vi "Find_Beam_Max_Pos.vi"(3 "Mode":T7, 5 "Traverse line In":T4 {"Row Duration (mins)" format="%#.1f"; "Row No" min=0; "Trace Gas Concentration (%)" min=0.0 format="%#.2f"; "Emission Rate (l/min)" format="%#.2f"; "Tunnel Speed" format="%#.2f"; "Start X" format="%#.2f"; "Start Y" format="%#.2f"; "Start Z" format="%#.2f"; "End X" format="%#.2f"; "End Y" format="%#.2f"; "End Z" format="%#.2f"; "Averaging time (min)" min=0.0 format="%#.2f"}) -> (0 "Error Message":string, 1 "Status":T3, 2 "Traverse line Out":T4 {"Row Duration (mins)" format="%#.1f"; "Row No" min=0; "Trace Gas Concentration (%)" min=0.0 format="%#.2f"; "Emission Rate (l/min)" format="%#.2f"; "Tunnel Speed" format="%#.2f"; "Start X" format="%#.2f"; "Start Y" format="%#.2f"; "Start Z" format="%#.2f"; "End X" format="%#.2f"; "End Y" format="%#.2f"; "End Z" format="%#.2f"; "Averaging time (min)" min=0.0 format="%#.2f"})   [LabVIEW 2012]
uses:
  Gen Trav/Traverse_cluster.ctl
  Gen Trav/Spacing.ctl
  Controls/Multi_run_mode.ctl
  Controls/User_Specific_mode.ctl
  Gen Trav/Multi_Run_Status.ctl
  Controls/Beam_Type.ctl
  Gen Trav/Route mapping/Axis.ctl
  ADAM Client/Sub VIs/ADAM Controls/Remember_value_mode.ctl
  Globals/Meas_global.vi
  Utilities/Email_transfer_global.vi
panel:
  out "Picture Log":path
  out "First Call":bool
  out "Fixed Axis":T1
  out "Beams to find":T2[](array[typedef]) items=["Green Unshifted", "Green Shifted", "Blue Unshifted", "Blue Shifted"]
  out "Beam Data":dbl[][](array[numeric]) format="%.2f"
  out "Beam Type":T2 items=["Green Unshifted", "Green Shifted", "Blue Unshifted", "Blue Shifted"]
  # "X                Y                 Z        Datum Power"
  # "Green Unshifted\nGreen Shifted\nBlue Unshifted\nBlue Shifted"
  # "X           Y            Z"
  # "Start"
  # "End"
  # "X           Y            Z"
  # "Start"
  # "End"
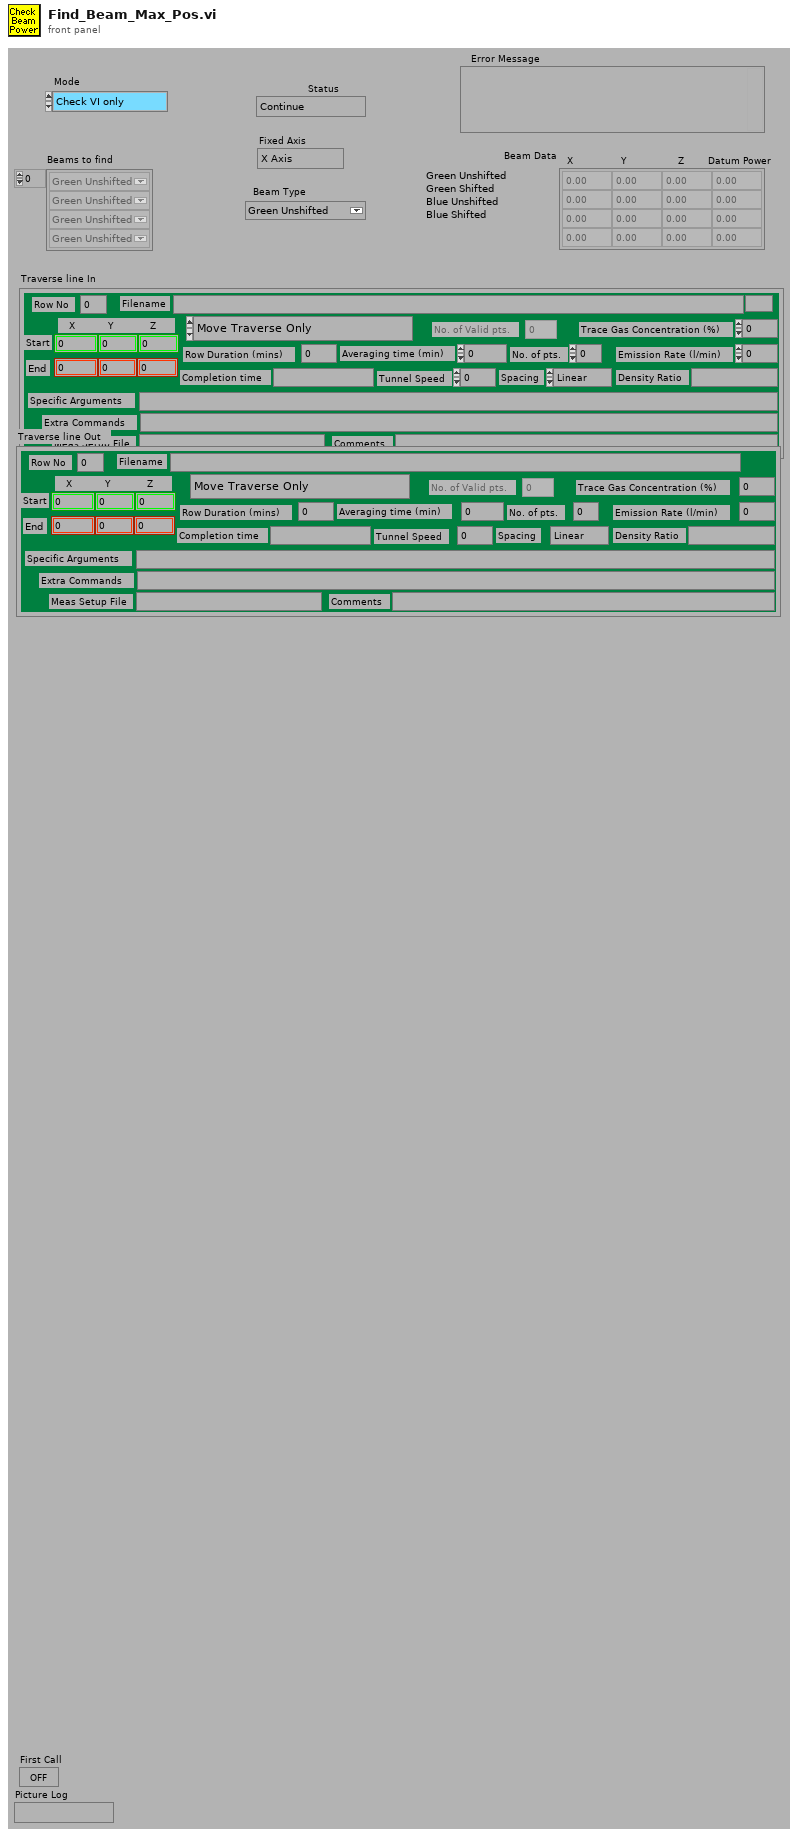
[diagram p1: front panel]
types:
  T1 = typedef "Axis.ctl" = enum16{"X Axis", "X Axis -ve", "Y Axis", "Y Axis -ve", "Z Axis", "Z Axis -ve"}
  T2 = typedef "Beam_Type.ctl" = u16
  T3 = typedef "Multi_Run_Status.ctl" = enum16{"Continue", "Jump to Next Point", "Jump to Next Row", "Jump To Fall Back", "Terminate Run"}
  T4 = typedef "Traverse_cluster.ctl" = cluster{"Start X":dbl, "Start Y":dbl, "Start Z":dbl, "End X":dbl, "End Y":dbl, "End Z":dbl, "No. of pts.":i32, "Spacing":T5, "Filename":path, "Tunnel Speed":dbl, "Averaging time (min)":dbl, "Extra Commands":string, "Specific Arguments":string, "Emission Rate (l/min)":dbl, "Trace Gas Concentration (%)":dbl, "Density Ratio":string, "Comments":string, "Row No":i32, "Row Type Selector":T6, "Completion time":string, "Row Duration (mins)":dbl, "No. of Valid pts.":i32, "Meas Setup File":string}
  T5 = typedef "Spacing.ctl" = enum16{"Linear", "Log", "Gauss", "Specified", "N/A"}
  T6 = typedef "Multi_run_mode.ctl" = enum16{"Move Traverse Only", "Set Tunnel Speed Only", "Set Source Only", "Set Measurement Conditions", "Single Measurement", "Vertical Profile", "Lateral Profile", "Longitudinal Profile", "Explore Volume", "Multi-Axis Profile", "Auto Calibrate", "Meas Fast FID Bkgnd", "Check Beam Power", "Scanning Valve Measurement", "Run VI Named:", "Set ADAM Ch", "Wait (minutes)", "Send Message", "Synchronize With:", "Fall Back to this Row", "Turn Off Row Repeating", "Blank Row", "Traverse 3D Volume"}
  T7 = typedef "User_Specific_mode.ctl" = enum16{"Check VI only", "Run VI"}
  T8 = typedef "LDA_Setup.ctl" = cluster{"dimensions":enum16{"1D", "2D"}, "Analogue Freq Multiplier":dbl}
  T9 = typedef "Remember_value_mode.ctl" = enum16{"Read only", "Read and Write"}
  T10 = enum16{"Load From Excel File", "Save to Excel File"}
  T11 = cluster{"second":i32, "minute":i32, "hour":i32, "day of month":i32, "month":i32, "year":i32, "day of week":i32, "day of year":i32, "is DST":i32}
  T12 = cluster{"path":path, "data":string, "binary":bool, "MIME content-type \n(application/octet-stream)":string}[]
  T13 = cluster{"path":path, "data":string, "binary":bool, "MIME content-type \n(application/octet-stream)":string}
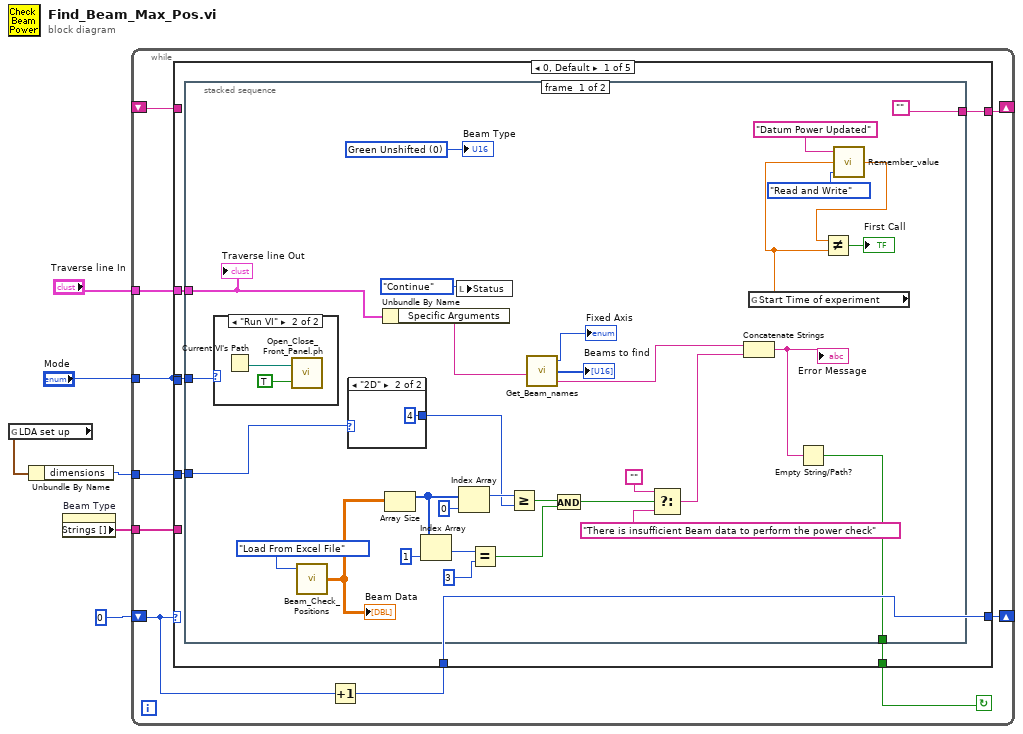
[diagram p0: block diagram]
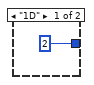
[diagram p2: hidden frame]
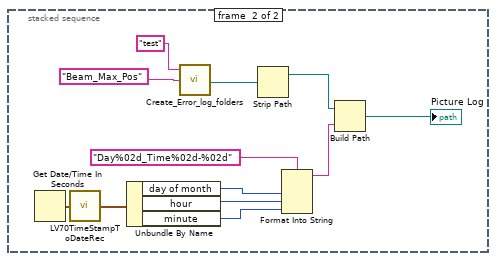
[diagram p4: hidden frame]
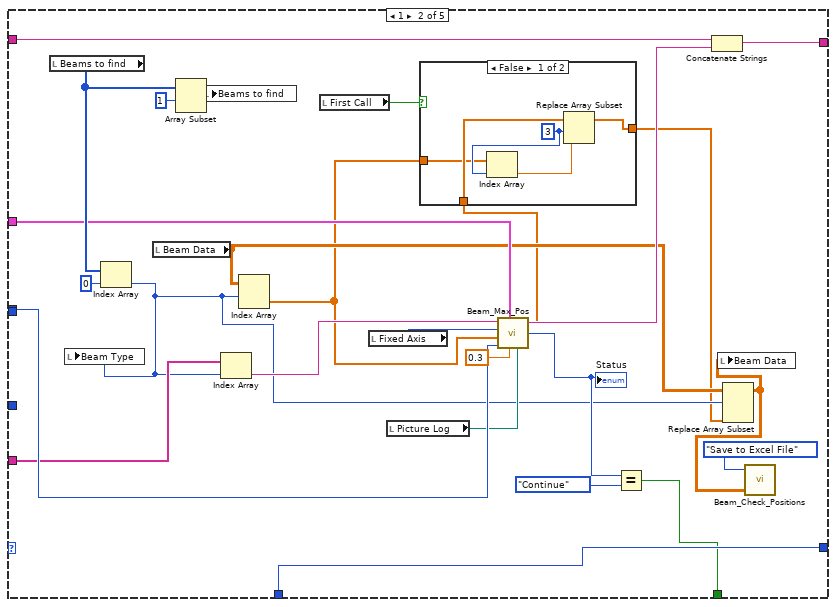
[diagram p5: hidden frame]
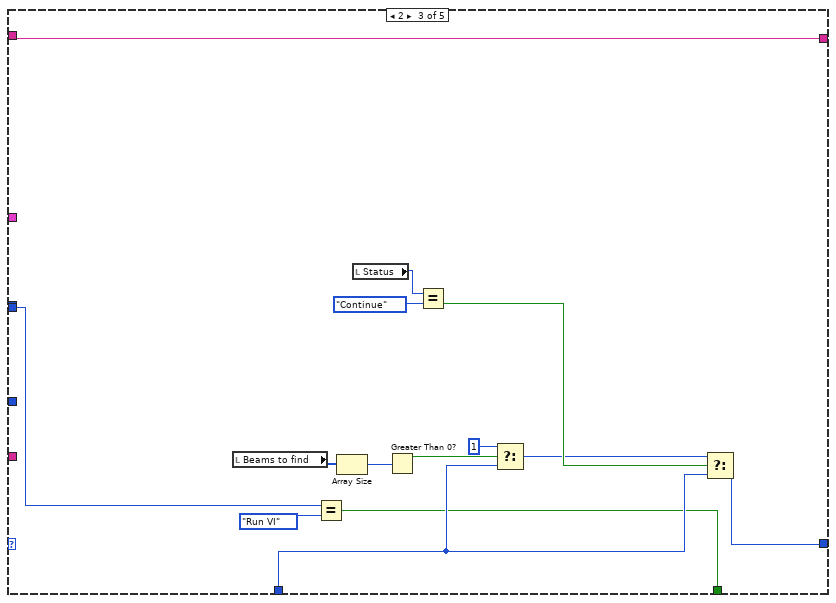
[diagram p7: hidden frame]
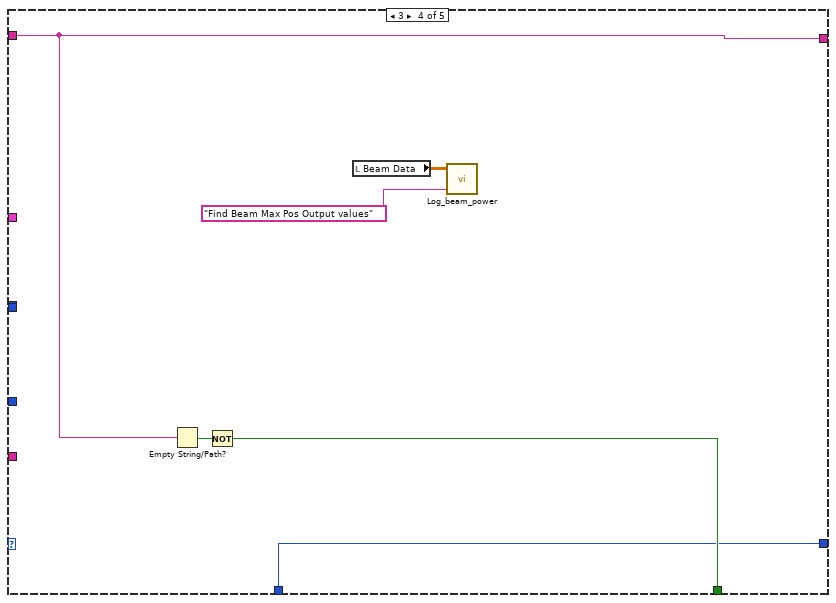
[diagram p8: hidden frame]
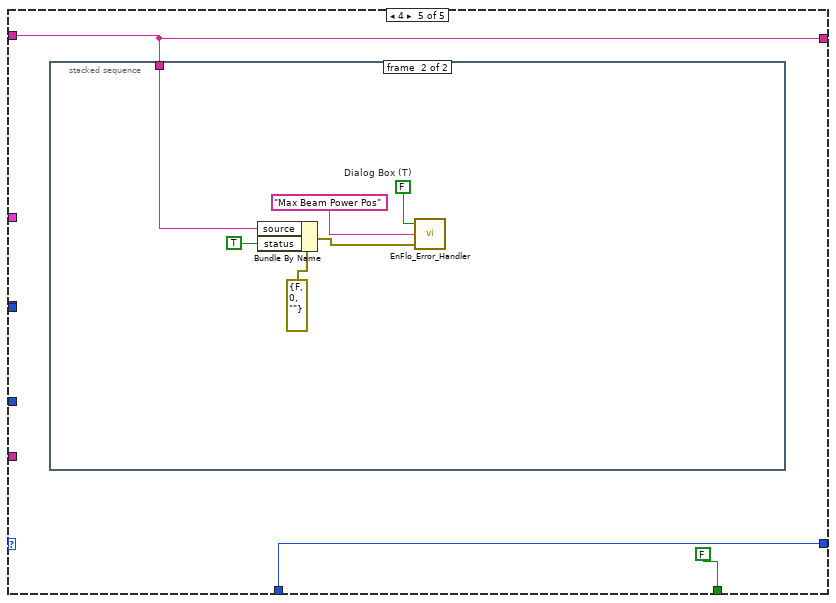
[diagram p9: hidden frame]
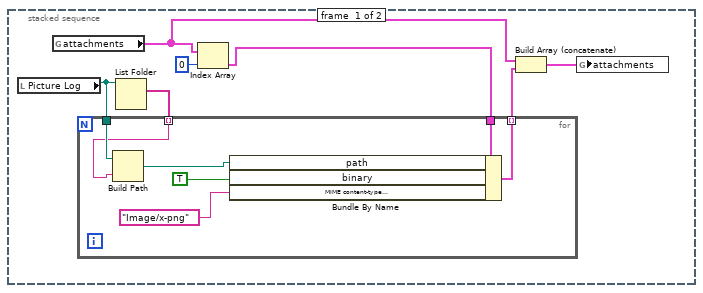
[diagram p10: hidden frame]
diagram:
  n1 = global read "Meas_global.vi" "LDA set up"() -> (w2:T8)
  n2 = Unbundle By Name(w2) -> ("dimensions"=w1:enum16{"1D", "2D"})
  n3 = property on="Beam Type" class="Ring (strict)"() -> ("Strings []"=w3:string[])  [unwired: 2 in, 2 out]
  n4 = while {
    shift-left: _ -> [w7]
    shift-right: [w8] -> _
    tunnel: w1 -> [w10]
    tunnel: w3 -> [w14]
    tunnel: "Traverse line In" -> [w15]
    tunnel: "Mode" -> [w9]
    shift-left: 0 -> [w16]
    shift-right: [w11] -> _
    stop <- w13 continue-if-true
    n5 = Increment(x=w16) -> (x+1=w12:i32)
    n6 = case shown="0, Default" w16 {
      tunnel: w15 -> [w18 w89 _ _ _]
      tunnel: w9 -> [w21 w90 _ _ _]
      tunnel: w14 -> [_ w81 _ _ _]
      tunnel: [w19 w83 w108 w118 FALSE] -> w13
      tunnel: w12 -> [w22 w92 w112 w117 w125]
      tunnel: [w22 w92 w111 w117 w125] -> w11
      tunnel: w10 -> [w20 _ _ _ _]
      tunnel: w9 -> [_ _ w109 _ _]
      tunnel: [w17 w86 w103 w120 w123] -> w8
      tunnel: w7 -> [_ w88 w103 w120 w123]
      frame 0, Default {
        n7 = stacked-sequence {
          tunnel: w21 -> [w49 _]
          tunnel: w20 -> [w48 _]
          tunnel: [w41 _] -> w19
          tunnel: w18 -> [w33 _]
          tunnel: ["" _] -> w17
          frame #0 {
            w53 = T2 0 items=["Green Unshifted", "Green Shifted", "Blue Unshifted", "Blue Shifted"] ("Beam Type")
            n8 = case shown="\"Run VI\"" w49 {
              frame "Check VI only" {
              }
              frame "Run VI" {
                n9 = Current VI's Path() -> (path=w57:path)
                n10 = call "Open_Close_Front_Panel.ph.vi"("Front Panel Window:Open"=TRUE, "VI path"=w57) -> ()  [unwired: 2 out]
              }
            }
            n11 = call "Beam_Check_Positions.vi"("Mode"=T10."Load From Excel File") -> ("Values Out"=w51:dbl[][])  [unwired: 1 in, 1 out]
            "Beam Data" <- w51
            n12 = case shown="\"2D\"" w48 {
              tunnel: [2 4] -> w46
              frame "1D" {
              }
              frame "2D" {
              }
            }
            n13 = Unbundle By Name(w33) -> ("Specific Arguments"=w23:string)
            n14 = Array Size(array=w51) -> (size(s)=w39:i32[])
            n15 = Index Array(array=w39, index=1 ("Index")) -> (element=w38:i32)
            n16 = local write "Status"(Multi_Run_Status."Continue" ("Status")) -> ()
            n17 = Index Array(array=w39, index=0 ("Index")) -> (element=w47:i32)
            n18 = Equal?(x=w38, y=3) -> (x = y?=w35:bool)
            n19 = Greater Or Equal?(x=w47, y=w46) -> (x >= y?=w36:bool)
            n20 = call "Get_Beam_names.vi"("String Value"=w23) -> ("Fixed Axis"=→"Fixed Axis":T1, "Beam Array"=→"Beams to find":T2[], "Error Comments"=w32:string)
            n21 = And(x=w36, y=w35) -> (x .and. y?=w34:bool)
            n22 = Select(t="", s=w34, f="There is insufficient Beam data to perform the power check") -> (s? t:f=w43:string)
            n23 = Concatenate Strings(w32, w43) -> (w42:string)
            "Error Message" <- w42
            n24 = global read "Meas_global.vi" "Start Time of experiment"() -> (w26:dbl)
            n25 = Empty String/Path?(string/path=w42) -> (empty?=w41:bool)
            n26 = call "Remember_value.vi"("Mode"=Remember_value_mode."Read and Write", "Input Value"=w26, "Ch name"="Datum Power Updated") -> ("Output Value"=w27:dbl)
            n27 = Not Equal?(x=w27, y=w26) -> (x != y?=→"First Call":bool)
            "Beam Type" <- w53
            "Traverse line Out" <- w33
          }
          frame #1 {
            n28 = Get Date/Time In Seconds() -> (seconds since 1Jan1904=w59:timestamp)
            n29 = call <vilib>:"LV70TimeStampToDateRec.vi"("time stamp"=w59) -> ("date time rec"=w68:T11)
            n30 = Unbundle By Name(w68) -> ("day of month"=w65:i32, "hour"=w66:i32, "minute"=w67:i32)
            n31 = call "Create_Error_log_folders.vi"("Log Folder"="Beam_Max_Pos" ("name or relative path"), "Log Filename"="test") -> ("Server copy Location"=w61:path)  [unwired: 1 in, 2 out]
            n32 = Strip Path(path=w61) -> (stripped path=w69:path)  [unwired: 1 out]
            n33 = Format Into String(format string="Day%02d_Time%02d-%02d", w65, w66, w67) -> (resulting string=w70:string)  [unwired: 2 in, 1 out]
            n34 = Build Path(base path=w69, name or relative path=w70) -> (appended path=→"Picture Log":path)
          }
        }
      }
      frame 1 {
        n35 = local read "Beams to find"() -> (w95:T2[])
        n36 = Index Array(array=w95, index=0 ("Index")) -> (element=w78:T2)
        n37 = local write "Beam Type"(w78) -> ()
        n38 = local read "Beam Data"() -> (w79:dbl[][])
        n39 = Array Subset(array=w95, index=1 ("Array Index")) -> (w93:T2[])  [unwired: 1 in]
        n40 = local write "Beams to find"(w93) -> ()
        n41 = Index Array(array=w81, index=w78) -> (element=w80:string)
        n42 = Index Array(array=w79, index (row)=w78) -> (element=w72:dbl[])  [unwired: 1 in]
        n43 = local read "First Call"() -> (w77:bool)
        n44 = local read "Fixed Axis"() -> (w91:T1)
        n45 = local read "Picture Log"() -> (w82:path)
        n46 = call "Beam_Max_Pos.vi"("Picture Log"=w82, "Search Step (mm)"=0.3, "Mode"=w90, "Starting Position"=w72, "Traverse line In"=w89, "Fixed Axis"=w91, "Beam Name"=w80) -> ("Status"=w84:T3, "Beam maxima"=w75:dbl[], "Message"=w87:string)  [unwired: 1 out]
        "Status" <- w84
        n47 = case shown="False" w77 {
          tunnel: [w100 w102] -> w76
          tunnel: w75 -> [w101 w102]
          tunnel: w72 -> [w98 _]
          frame False {
            w99 = 3 ("index")
            n48 = Index Array(array=w98, index=w99) -> (element=w97:dbl)
            n49 = Replace Array Subset(array=w101, new element=w97, index=w99) -> (w100:dbl[])
          }
          frame True {
          }
        }
        n50 = Equal?(x=w84, y=Multi_Run_Status."Continue" ("Status")) -> (x = y?=w83:bool)
        n51 = Concatenate Strings(w88, w87) -> (w86:string)
        n52 = Replace Array Subset(array=w79, new element=w76, index (row)=w78) -> (w73:dbl[][])  [unwired: 1 in]
        n53 = local write "Beam Data"(w73) -> ()
        n54 = call "Beam_Check_Positions.vi"("Values"=w73, "Mode"=T10."Save to Excel File") -> ()  [unwired: 2 out]
      }
      frame 2 {
        n55 = local read "Beams to find"() -> (w107:T2[])
        n56 = Equal?(x=w109, y=User_Specific_mode."Run VI" ("Mode")) -> (x = y?=w108:bool)
        n57 = Array Size(array=w107) -> (size(s)=w106:i32)
        n58 = local read "Status"() -> (w116:T3)
        n59 = Greater Than 0?(x=w106) -> (x > 0?=w105:bool)
        n60 = Equal?(x=w116, y=Multi_Run_Status."Continue" ("Status")) -> (x = y?=w114:bool)
        n61 = Select(t=1, s=w105, f=w112) -> (s? t:f=w113:i32)
        n62 = Select(t=w113, s=w114, f=w112) -> (s? t:f=w111:i32)
      }
      frame 3 {
        n63 = Empty String/Path?(string/path=w120) -> (empty?=w119:bool)
        n64 = Not(x=w119) -> (.not. x?=w118:bool)
        n65 = local read "Beam Data"() -> (w122:dbl[][])
        n66 = call "Log_beam_power.vi"("Message"="Find Beam Max Pos Output values", "Beam Data"=w122) -> ()  [unwired: 4 out]
      }
      frame 4 {
        n67 = stacked-sequence {
          tunnel: w123 -> [_ w140]
          frame #0 {
            n68 = local read "Picture Log"() -> (w127:path)
            n69 = global read "Email_transfer_global.vi" "attachments"() -> (w130:T12)
            n70 = List Folder(path=w127) -> (filenames=w126:string[])  [unwired: 1 in, 5 out]
            n71 = Index Array(array=w130, index=0) -> (element=w129:T13)
            n72 = for {
              tunnel: [w137] -> w132 mode=indexing
              tunnel: w129 -> [w136]
              tunnel: w127 -> [w135]
              tunnel: w126 -> [w134] mode=indexing
              n73 = Build Path(base path=w135, name or relative path=w134) -> (appended path=w133:path)
              n74 = Bundle By Name(cluster=w136, "path"=w133, "binary"=TRUE, "MIME content-type \n(application/octet-stream)"="Image/x-png" ("MIME content-type \n(application/octet-stream)")) -> (w137:T13)
            }
            n75 = Build Array (concatenate)(w130, w132) -> (w131:T12)
            n76 = global write "Email_transfer_global.vi" "attachments"(w131) -> ()
          }
          frame #1 {
            w144 = FALSE  # Dialog Box (T)
            n77 = Bundle By Name(cluster=errorcluster {"status"=FALSE, "code"=0, "source"=""} ("error in (no error)"), "source"=w140, "status"=TRUE ("Bundle Element")) -> (w142:errorcluster)
            n78 = call "EnFlo_Error_Handler.vi"("error in (no error)"=w142, "Error Type"="Max Beam Power Pos", "Dialog Box (T)"=w144) -> ()  [unwired: 3 out]
          }
        }
      }
    }
  }
